vi "Read Waveform.vi"(8 "error in (no error)":errorcluster, 10 "Parameters 3":T1={"Source (0: Channel 1)"=0, "Timeout (10000 ms)"=10000} {"Source (0: Channel 1)" items=["Channel 1", "Channel 2", "Channel 3", "Channel 4", "Math", "Reference A", "Reference B", "Reference C", "Reference D", "FFT"]}, 11 "Tektonix 2000 in":refnum<class "Tektonix 2000.lvclass">) -> (0 "error out":errorcluster, 2 "Waveform Data":waveform(dbl)(graph), 3 "Tektonix 2000 out":refnum<class "Tektonix 2000.lvclass">)   [LabVIEW 2020, in "Osciloscope Tektronix.lvlib" / "Tektonix 2000.lvclass"]
uses:
  Tektonix 2000.lvclass
  C:/Users/Pablo/Osciloscope-Tek/TDS2000/Libraries/Osciloscope Tektronix/Clases/Osciloscope/Osciloscope.lvclass
  Osciloscope/Osciloscope.lvclass/Osciloscope.ctl
  Osciloscope/Read COM.vi
  Osciloscope/Read Probe Attenuation.vi
  <instrlib>/Tektronix TDS 200 1000 2000 Series/Public/Data/Read (Single Waveform).vi
  <instrlib>/Tektronix TDS 200 1000 2000 Series/Tektronix TDS 200 1000 2000 Series.lvlib
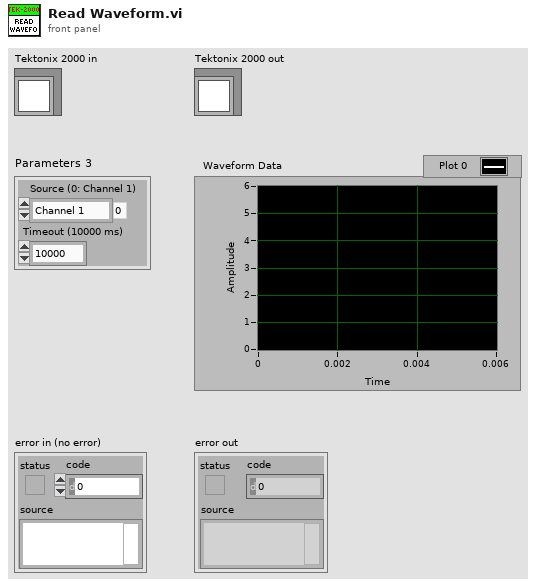
[diagram p1: front panel]
types:
  T1 = cluster{"Source (0: Channel 1)":u16, "Timeout (10000 ms)":u32}
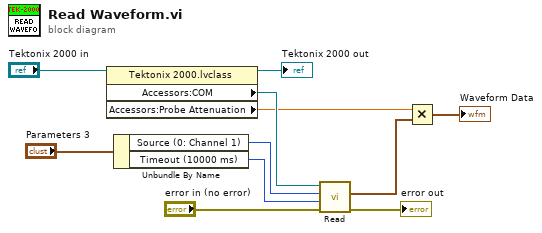
[diagram p0: block diagram]
diagram:
  n1 = property class="Tektonix 2000.lvclass"(reference="Tektonix 2000 in") -> (reference out=→"Tektonix 2000 out":refnum<class "Tektonix 2000.lvclass">, "Accessors:COM"=w9:refnum<visa-resource-name>, "Accessors:Probe Attenuation"=w3:dbl)  [unwired: 1 in, 1 out]
  n2 = Unbundle By Name("Parameters 3") -> ("Source (0: Channel 1)"=w5:u16, "Timeout (10000 ms)"=w4:u32)
  n3 = call-poly <instrlib>:"Read.vi"("error in (no error)"="error in (no error)", "Timeout (10000 ms)"=w4, "Source (0: Channel 1)"=w5, "VISA resource name"=w9) -> ("error out"=→"error out":errorcluster, "Waveform Data"=w2:waveform(dbl))  [unwired: 5 in, 1 out]
  n4 = Multiply(x=w3, y=w2) -> (x*y=→"Waveform Data":waveform(dbl))
